vi "Mainframe_VISAs(gbl).vi"() -> ()   [LabVIEW 2018]
panel:
  in  "Mainframe 2 VISA":refnum<visa-resource-name>
  in  "Mainframe 1 VISA":refnum<visa-resource-name>
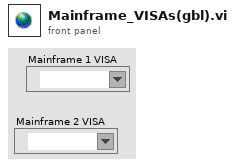
[diagram p1: front panel]
diagram:
